vi "DSF.Engine.Memory.Cache.Plugin.Create.vi"(7 "Transfer Group Cache type":refnum<class "DSF.Engine.Memory.Cache.Transfer Group.lvclass">, 8 "error in (no error)":errorcluster, 10 "Plugin Configuration":refnum<class "DSF.Shared.Configuration.Plugin.lvclass">, 11 "Plugin Cache type":refnum<class "DSF.Engine.Memory.Cache.Plugin.lvclass">) -> (0 "error out":errorcluster, 3 "Plugin Cache":refnum<class "DSF.Engine.Memory.Cache.Plugin.lvclass">)   [LabVIEW 2016, in "DSF.Engine.lvlib" / "DSF.Engine.Memory.Cache.Plugin.lvclass"]
uses:
  DSF.Engine.Memory.Cache.Plugin.lvclass
  DSF.Engine.Memory.Cache.Transfer Group.lvclass
  Shared/Classes/Plugin/DSF.Shared.Configuration.Plugin.lvclass
  Shared/Classes/Plugin/DSF.Shared.Configuration.Plugin.lvclass/DSF.Shared.Configuration.Plugin.ctl
  DSF.Engine.Memory.Cache.Plugin.lvclass/DSF.Engine.Memory.Cache.Plugin.ctl
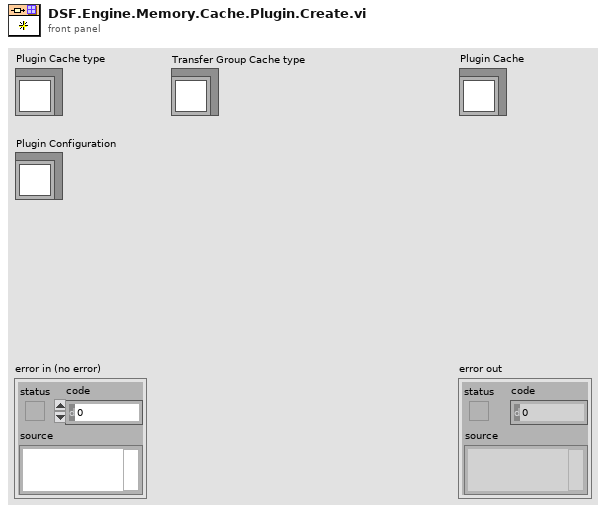
[diagram p1: front panel]
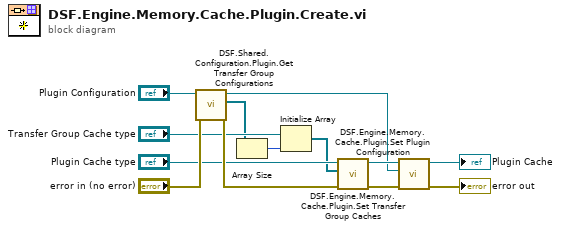
[diagram p0: block diagram]
diagram:
  n1 = call "DSF.Shared.Configuration.Plugin.Get Transfer Group Configurations.vi"("error in (no error)"="error in (no error)", "Plugin Configuration in"="Plugin Configuration") -> ("error out"=w13:errorcluster, "Transfer Group Configurations"=w3:refnum<class "DSF.Shared.Configuration.Transfer Group.lvclass">[], "Plugin Configuration out"=w5:refnum<class "DSF.Shared.Configuration.Plugin.lvclass">)  [unwired: 7 in]
  n2 = Array Size(array=w3) -> (size(s)=w11:i32)
  n3 = Initialize Array("Transfer Group Cache type", w11) -> (w4:refnum<class "DSF.Engine.Memory.Cache.Transfer Group.lvclass">[])
  n4 = call "DSF.Engine.Memory.Cache.Plugin.Set Transfer Group Caches.vi"("error in (no error)"=w13, "Transfer Group Caches"=w4, "Plugin Cache in"="Plugin Cache type") -> ("error out"=w7:errorcluster, "Plugin Cache out"=w6:refnum<class "DSF.Engine.Memory.Cache.Plugin.lvclass">)  [unwired: 7 in]
  n5 = call "DSF.Engine.Memory.Cache.Plugin.Set Plugin Configuration.vi"("error in (no error)"=w7, "Plugin Configuration"=w5, "Plugin Cache in"=w6) -> ("error out"=→"error out":errorcluster, "Plugin Cache out"=→"Plugin Cache":refnum<class "DSF.Engine.Memory.Cache.Plugin.lvclass">)  [unwired: 7 in]
